vi "Point-in-Tri test.vi"(1 "Point":sgl[](array[numeric]), 2 "Triangle":T1) -> (0 "Point is inside triangle":bool)   [LabVIEW 2014]
uses:
  Typedefs/Triangle.ctl
panel:
  # "PN 13/01/2015"
  # "Vertices"
  # "Edges"
  # "Unit normal"
  # "pre-store"
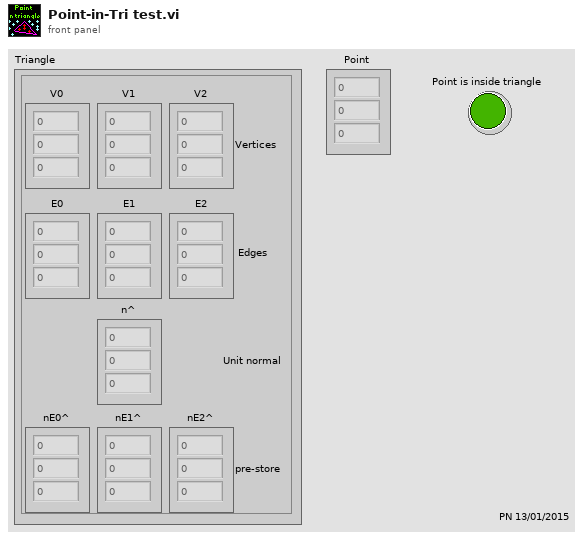
[diagram p1: front panel]
types:
  T1 = typedef "Triangle.ctl" = cluster{"V0":sgl[], "V1":sgl[], "V2":sgl[], "E0":sgl[], "E1":sgl[], "E2":sgl[], "n^":sgl[], "nE0^":sgl[], "nE1^":sgl[], "nE2^":sgl[]}
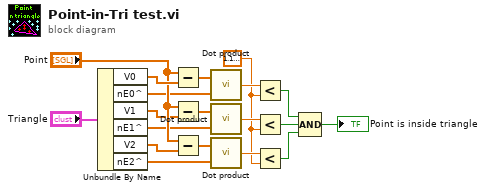
[diagram p0: block diagram]
diagram:
  w5 = sgl 1.1920929e-07
  n1 = Unbundle By Name("Triangle") -> ("V0"=w18:sgl[], "nE0^"=w9:sgl[], "V1"=w10:sgl[], "nE1^"=w11:sgl[], "V2"=w13:sgl[], "nE2^"=w12:sgl[])
  n2 = Subtract(x="Point", y=w18) -> (x-y=w16:sgl[])
  n3 = Subtract(x="Point", y=w10) -> (x-y=w14:sgl[])
  n4 = Subtract(x="Point", y=w13) -> (x-y=w15:sgl[])
  n5 = call "Dot product.vi"("B"=w9, "A"=w16) -> ("A . B"=w8:sgl)
  n6 = call "Dot product.vi"("B"=w11, "A"=w14) -> ("A . B"=w7:sgl)
  n7 = call "Dot product.vi"("B"=w12, "A"=w15) -> ("A . B"=w6:sgl)
  n8 = Less?(x=w8, y=w5) -> (x < y?=w4:bool)
  n9 = Less?(x=w7, y=w5) -> (x < y?=w3:bool)
  n10 = Less?(x=w6, y=w5) -> (x < y?=w2:bool)
  n11 = Compound Arithmetic op=AND(w4, w3, w2) -> (→"Point is inside triangle":bool)
